vi "Thread Loop.vi"(8 "error in (no error)":errorcluster, 11 "Wash Display Console in":refnum<class "Wash Display Console.lvclass">) -> (0 "error out":errorcluster, 3 "Wash Display Console out":refnum<class "Wash Display Console.lvclass">)   [LabVIEW 2019, in "Wash Display Console.lvlib" / "Wash Display Console.lvclass"]
uses:
  Wash Display Console.lvclass
  Thread/Thread.lvclass
  Entry Console/Wash Step Indicators.ctl
panel:
  out "Time Remaining":string
  out "Vehicle Out of Position":bool
  out "Wash Step Indicators":T1={"Blank Button"=FALSE, "Blank Button 2"=FALSE, "Blank Button 3"=FALSE, "Blank Button 4"=TRUE, "Blank Button 5"=FALSE, "Blank Button 6"=FALSE, "Blank Button 7"=FALSE, "Blank Button 8"=FALSE}
  out "Wash Entry":string
  # "[Covers: UI3]"
  # "[Covers: UI3A]"
  # "[Covers: UI3B]"
  # "[Covers: UI3B1]"
  # "[Covers: UI3C]"
  # "[Covers: UI3D]"
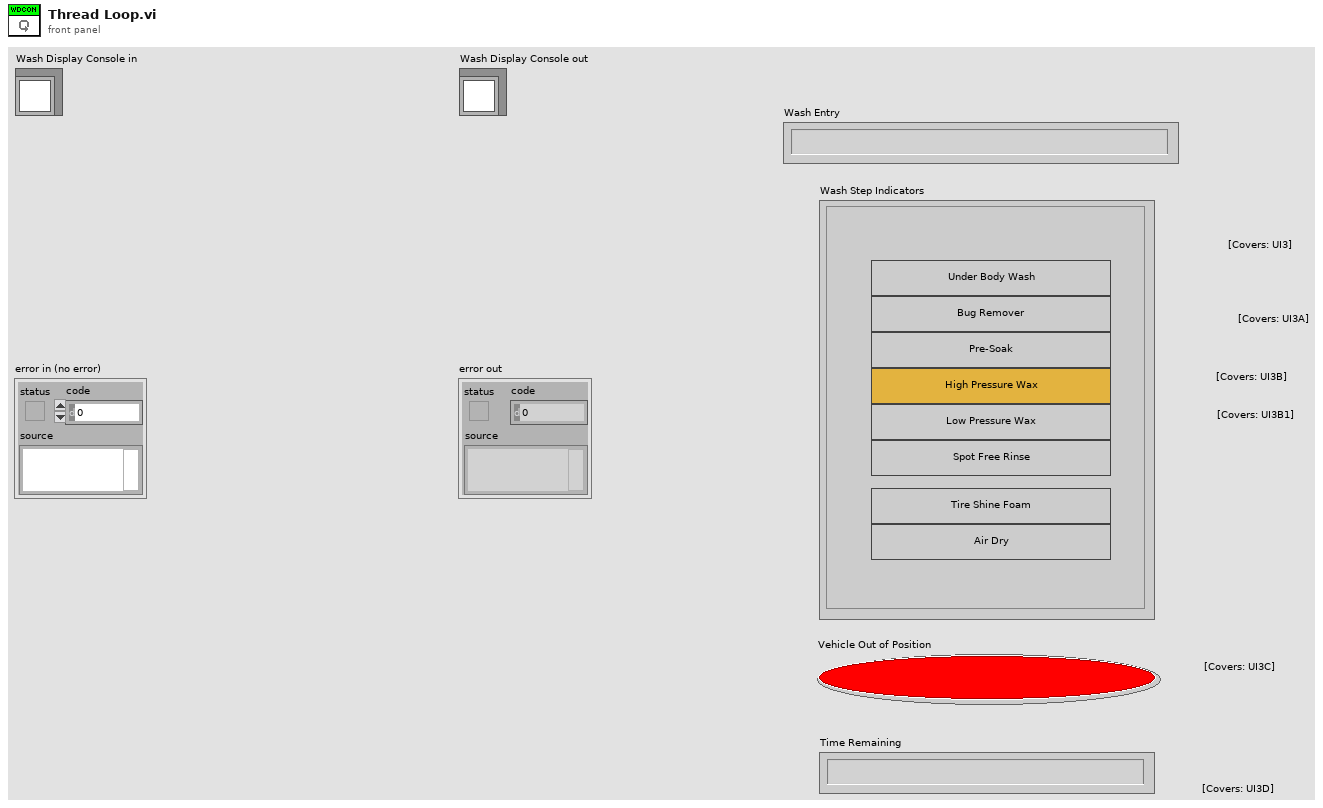
[diagram p1: front panel]
types:
  T1 = typedef "Wash Display Console.lvlib/Wash Display Console.lvclass/Wash Step Indicators.ctl" = cluster{"Blank Button":bool, "Blank Button 2":bool, "Blank Button 3":bool, "Blank Button 4":bool, "Blank Button 5":bool, "Blank Button 6":bool, "Blank Button 7":bool, "Blank Button 8":bool}
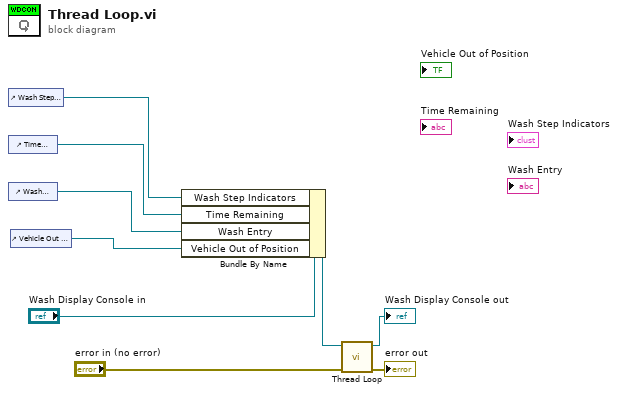
[diagram p0: block diagram]
diagram:
  n1 = control-ref of="Wash Step Indicators"() -> (w4:refnum<vi>)
  n2 = control-ref of="Time Remaining"() -> (w3:refnum<vi>)
  n3 = control-ref of="Wash Entry"() -> (w2:refnum<vi>)
  n4 = control-ref of="Vehicle Out of Position"() -> (w1:refnum<vi>)
  n5 = Bundle By Name(cluster="Wash Display Console in", "Wash Step Indicators"=w4, "Time Remaining"=w3, "Wash Entry"=w2, "Vehicle Out of Position"=w1) -> (w5:refnum<class "Wash Display Console.lvclass">)
  n6 = call-parent "Thread Loop.vi"("error in (no error)"="error in (no error)", "Thread in"=w5) -> ("error out"=→"error out":errorcluster, "Thread out"=→"Wash Display Console out":refnum<class "Wash Display Console.lvclass">)  [unwired: 8 in]
